vi "Host-Top-Level-Chirp-FFT-PowerSpectrum.vi"(8 "error in":errorcluster, 11 "Run Number\nto Load":i32=1) -> (3 "PowerSpectrum":dbl[][](array[numeric]))   [LabVIEW 2015, in "SETI_LV.lvlib"]
uses:
  SETI_LV.lvlib
  <vilib>/Analysis/2dsp.llb/Complex FFT.vi
  <vilib>/Analysis/NI_AALPro.lvlib
panel:
  out "binWorkUnitDataPoints.bin (DataIn) out":csg[][](array[numeric])
  out "FFT {X}":cdb[][](array[numeric])
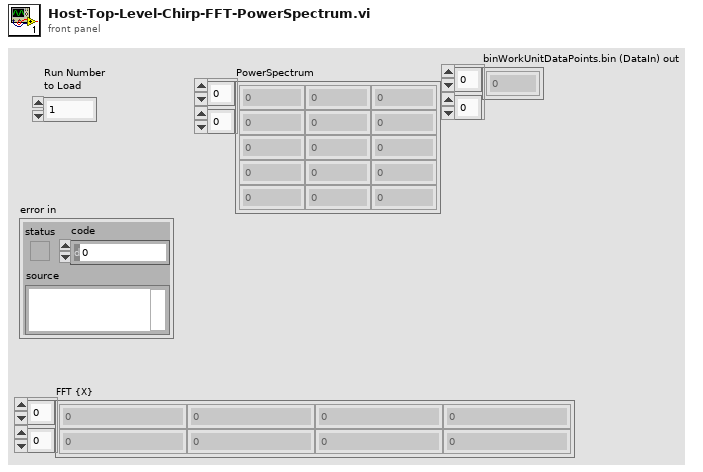
[diagram p1: front panel]
types:
  T1 = typedef "SETI_LV.lvlib/ChirpFFT Pairs.ctl" = cluster{"Chirp/Fft Pair 1 - Chirp Rate":dbl, "Chirp/Fft Pair 1 - Chirp Rate Ind":i32, "Chirp/Fft Pair 1 - Fft Length":i32, "Chirp/Fft Pair 1 - Pulse Find":i32, "Chirp/Fft Pair 1 - Gauss Fit":i32}
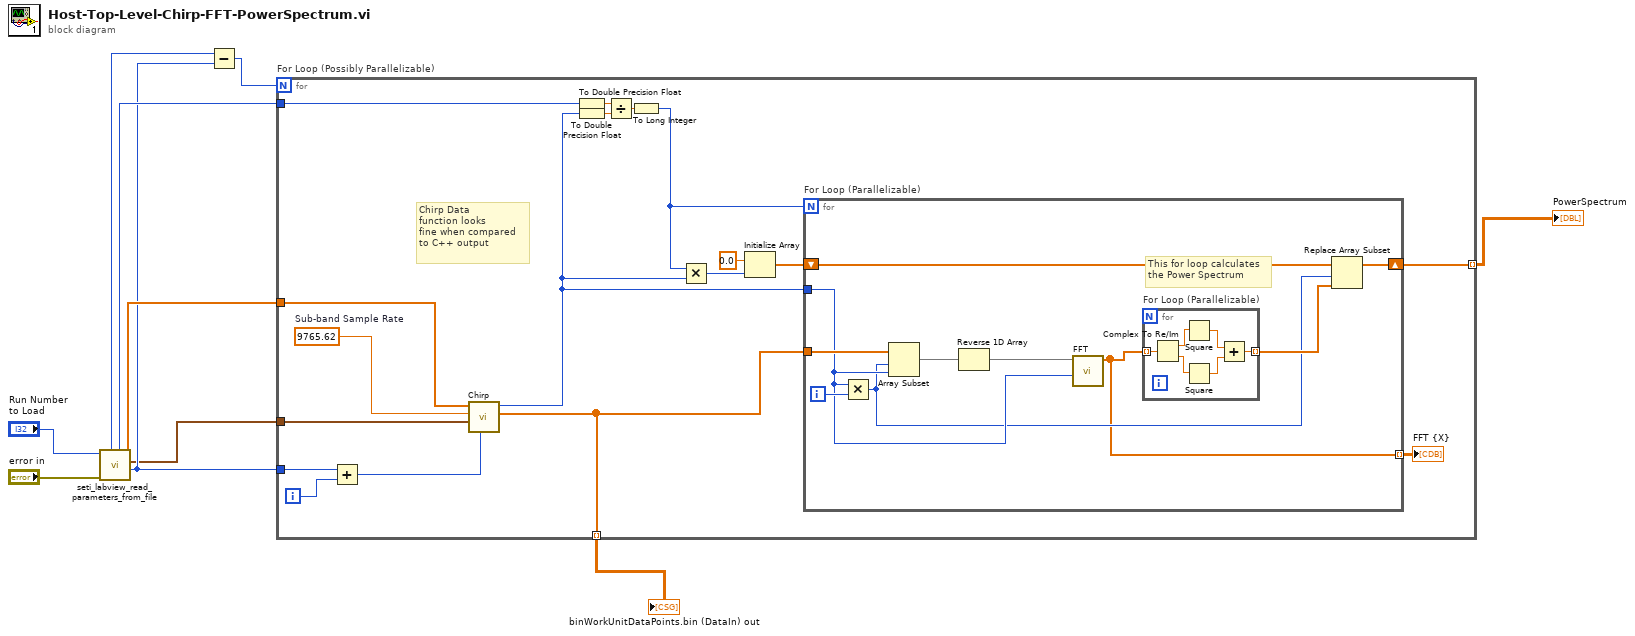
[diagram p0: block diagram]
diagram:
  n1 = call "seti_labview_read_parameters_from_file.vi"("error in (no error)"="error in", "Run Number\nto Load"="Run Number\nto Load") -> ("start_icfft"=w4:i32, "Chirp FFT Pairs"=w3:T1[], "Data Points (Source)"=w10:csg[], "NumDataPoints"=w9:u32, "end_icfft"=w5:i32)  [unwired: 3 in, 2 out]
  n2 = Subtract(x=w5, y=w4) -> (x-y=w7:i32)
  n3 = for "For Loop (Possibly Parallelizable)" {
    N: w7 -> [_]
    tunnel: w4 -> [w28]
    tunnel: w3 -> [w27]
    tunnel: w10 -> [w26]
    tunnel: w9 -> [w24]
    tunnel: [w17] -> w6 mode=indexing
    tunnel: [w11] -> w1 mode=indexing
    i -> [w22]
    w25 = 9765.62  # Sub-band Sample Rate
    # "Chirp Data\nfunction looks\nfine when compared\nto C++ output"
    n4 = Add(x=w28, y=w22) -> (x+y=w15:i32)
    n5 = call "Chirp.vi"("icfft"=w15, "Chirp FFT Pairs"=w27, "Sub-band Sample Rate"=w25, "binWorkUnitDataPoints.bin (DataIn) in"=w26) -> ("binWorkUnitDataPoints.bin (DataIn) out"=w11:csg[], "Chirp/Fft Pair 1 - Fft Length"=w16:i32)  [unwired: 1 in, 5 out]
    n6 = To Double Precision Float(number=w24) -> (double precision float=w21:dbl)
    n7 = To Double Precision Float(number=w16) -> (double precision float=w20:dbl)
    n8 = Divide(x=w21, y=w20) -> (x/y=w23:dbl)
    n9 = To Long Integer(number=w23) -> (32bit integer=w18:i32)
    n10 = Multiply(x=w18, y=w16) -> (x*y=w13:i32)
    n11 = Initialize Array(0.0, w13) -> (w14:dbl[])
    n12 = for "For Loop (Parallelizable)" {
      N: w18 -> [_]
      tunnel: w11 -> [w38]
      tunnel: w16 -> [w33]
      shift-right: [w35] -> w17
      shift-left: w14 -> [w36]
      tunnel: [w29] -> w12 mode=indexing
      i -> [w37]
      # "This for loop calculates\nthe Power Spectrum"
      n13 = Multiply(x=w33, y=w37) -> (x*y=w32:i32)
      n14 = Array Subset(array=w38, index=w32, length=w33) -> (w31:csg[])
      n15 = Reverse 1D Array(array=w31) -> (reversed array=w30:csg[])
      n16 = call-poly <vilib>:"FFT.vi"("FFT size"=w33, "X"=w30) -> ("FFT {X}"=w29:cdb[])  [unwired: 8 in, 1 out]
      n17 = for "For Loop (Parallelizable)" {
        tunnel: w29 -> [w44] mode=indexing
        tunnel: [w41] -> w34 mode=indexing
        n18 = Complex To Re/Im(x + iy=w44) -> (x=w43:dbl, y=w42:dbl)
        n19 = Square(x=w43) -> (x^2=w40:dbl)
        n20 = Square(x=w42) -> (x^2=w39:dbl)
        n21 = Add(x=w40, y=w39) -> (x+y=w41:dbl)
      }
      n22 = Replace Array Subset(array=w36, new element=w34, index=w32) -> (w35:dbl[])
    }
    "FFT {X}" <- w12
  }
  "PowerSpectrum" <- w6
  "binWorkUnitDataPoints.bin (DataIn) out" <- w1
